vi "Write Text Width.vi"(5 "Text Width":u32, 9 "Digital in":refnum<class "Digital.lvclass">) -> (3 "Digital out":refnum<class "Digital.lvclass">)   [LabVIEW 2014, in "Raspberry Pi Compatible Compiler for LabVIEW.lvlib" / "Digital.lvclass"]
uses:
  Digital.lvclass
  Digital.lvclass/Digital.ctl
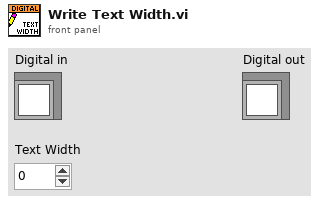
[diagram p1: front panel]
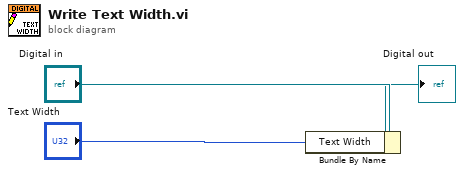
[diagram p0: block diagram]
diagram:
  n1 = Bundle By Name(cluster="Digital in", "Text Width"="Text Width") -> (→"Digital out":refnum<class "Digital.lvclass">)
